vi "06-5-Save B-Scans To Disk.vi"(8 "Enable Logging?":bool, 9 "DVR Test 2":refnum<data-value>, 10 "DVR Test 1":refnum<data-value>, 11 "B-Scan Finished?":bool) -> (1 "DVR Test 2 out":refnum<data-value>, 2 "DVR Test 1 out":refnum<data-value>)   [LabVIEW 2026]
uses:
  <vilib>/Utility/file.llb/Write Delimited Spreadsheet (I64).vi
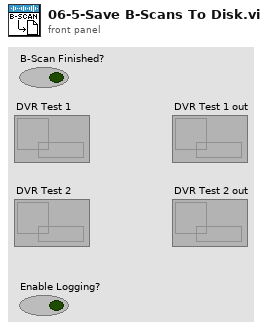
[diagram p1: front panel]
types:
  T1 = enum16{"open", "replace", "create", "open or create", "replace or create", "replace or create with confirmation"}
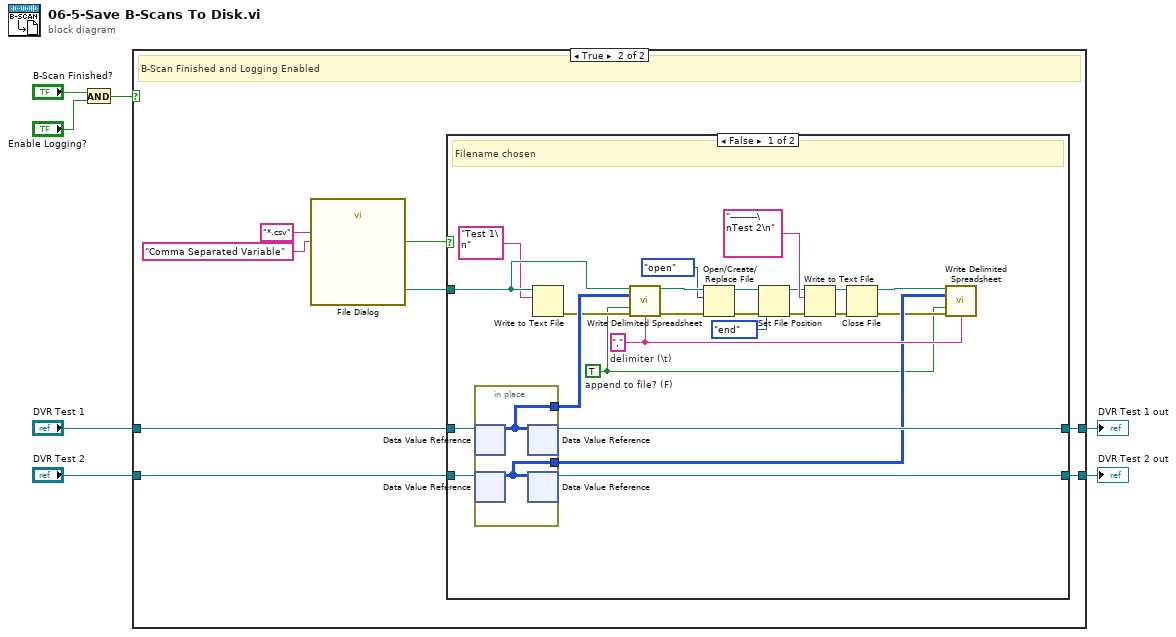
[diagram p0: block diagram]
diagram:
  n1 = And(x="B-Scan Finished?", y="Enable Logging?") -> (x .and. y?=w6:bool)
  n2 = case shown="True" w6 {
    tunnel: "DVR Test 1" -> [w9 w13]
    tunnel: "DVR Test 2" -> [w8 w12]
    tunnel: [w9 w11] -> w2
    tunnel: [w8 w10] -> w1
    frame False {
      # "Do Nothing"
    }
    frame True {
      # "B-Scan Finished and Logging Enabled"
      n3 = call "File Dialog"("pattern (all files)"="*.csv", "pattern label"="Comma Separated Variable") -> ("selected path"=w14:path, "cancelled"=w15:bool)  [unwired: 10 in, 2 out]
      n4 = case shown="False" w15 {
        tunnel: w14 -> [w20 _]
        tunnel: w13 -> [w39 w43]
        tunnel: w12 -> [w38 w42]
        tunnel: [w37 w43] -> w11
        tunnel: [w36 w42] -> w10
        frame False {
          w18 = TRUE  # append to file? (F)
          w30 = ","  # delimiter (\t)
          # "Filename chosen"
          n5 = in-place {
            in-place-border: [w41] -> w35
            in-place-border: [w40] -> w25
            n6 = in-place-dvr #1(w39) -> (w41:u16[][])  [unwired: 1 out]
            n7 = in-place-dvr #2(w38) -> (w40:u16[][])  [unwired: 1 out]
            n8 = in-place-dvr #1(w41) -> (w37:refnum<data-value>)  [unwired: 1 out]
            n9 = in-place-dvr #2(w40) -> (w36:refnum<data-value>)  [unwired: 1 out]
          }
          n10 = Write to Text File(file (use dialog)=w20, text="Test 1\n") -> (error out=w21:errorcluster)  [unwired: 2 in, 2 out]
          n11 = call-poly <vilib>:"Write Delimited Spreadsheet.vi"("file path (dialog if empty)"=w20, "2D data"=w35, "append to file? (new file:F)"=w18, "error in (no error)"=w21, "delimiter (\\t)"=w30) -> ("new file path (Not A Path if cancelled)"=w31:path, "error out"=w34:errorcluster)  [unwired: 9 in]
          n12 = Open/Create/Replace File(file path (use dialog)=w31, operation (0:open)=T1."open") -> (refnum out=w29:refnum<file>)  [unwired: 4 in, 2 out]
          n13 = Set File Position(refnum=w29, from (0:start)=enum16{"start", "end", "current"}."end") -> (refnum out=w27:refnum<file>)  [unwired: 2 in, 1 out]
          n14 = Write to Text File(file (use dialog)=w27, text="---------\nTest 2\n", error in=w34) -> (refnum out=w23:refnum<file>, error out=w32:errorcluster)  [unwired: 1 in, 1 out]
          n15 = Close File(refnum=w23, error in=w32) -> (path=w22:path, error out=w24:errorcluster)
          n16 = call-poly <vilib>:"Write Delimited Spreadsheet.vi"("file path (dialog if empty)"=w22, "2D data"=w25, "append to file? (new file:F)"=w18, "error in (no error)"=w24, "delimiter (\\t)"=w30) -> ()  [unwired: 9 in, 2 out]
        }
        frame True {
          # "Cancelled - Do Nothing"
        }
      }
    }
  }
  "DVR Test 2 out" <- w1
  "DVR Test 1 out" <- w2
